vi "Get Kasli IP.vi"(8 "error in (no error)":errorcluster, 11 "Kasli Writer in":refnum<class "Kasli Writer.lvclass">) -> (0 "error out":errorcluster, 3 "Kasli Writer out":refnum<class "Kasli Writer.lvclass">)   [LabVIEW 2020, in "CIRCUS_uServices.lvlib" / "Kasli Listener and Writer.lvlib" / "Kasli Writer.lvclass"]
uses:
  Kasli Writer.lvclass
  C:/Users/marco/Documents/GitHub_Lab/CIRCUS/TALOS/TALOS_PPL.lvlibp/Ancestor/Ancestor/Ancestor.lvclass
  C:/Users/marco/Documents/GitHub_Lab/CIRCUS/TALOS/TALOS_PPL.lvlibp/Internal uServices/System uServices/TCP Writer/TCP Writer/TCP Writer.lvclass
  TALOS/TALOS_PPL.lvlibp/Ancestor/Ancestor/Read ID.vi
  TALOS/TALOS_PPL.lvlibp
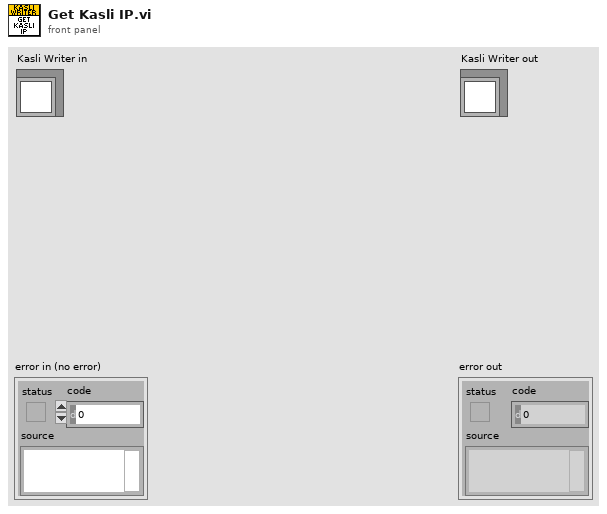
[diagram p1: front panel]
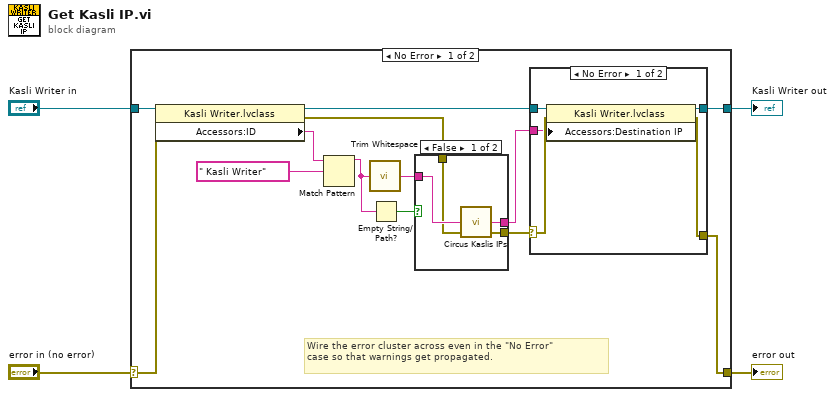
[diagram p0: block diagram]
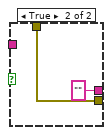
[diagram p3: hidden frame]
diagram:
  n1 = case shown="No Error" "error in (no error)" {
    selector: "error in (no error)" -> [w9 w32]
    tunnel: [w5 w32] -> w3
    tunnel: [w8 w31] -> w1
    tunnel: "Kasli Writer in" -> [w17 w31]
    frame No Error {
      # "Wire the error cluster across even in the \"No Error\"\ncase so that warnings get propagated."
      n2 = property class="Kasli Writer.lvclass"(reference=w17, error in=w9) -> (reference out=w16:refnum<class "Kasli Writer.lvclass">, error out=w10:errorcluster, "Accessors:ID"=w15:string)
      n3 = Match Pattern(string=w15, regular expression=" Kasli Writer") -> (before substring=w11:string)  [unwired: 1 in, 3 out]
      n4 = call <vilib>:"Trim Whitespace.vi"("string"=w11) -> ("trimmed string"=w12:string)  [unwired: 1 in]
      n5 = Empty String/Path?(string/path=w11) -> (empty?=w13:bool)
      n6 = case shown="False" w13 {
        tunnel: w12 -> [w28 _]
        tunnel: [w26 "" ("IP")] -> w7
        tunnel: [w25 w29] -> w6
        tunnel: w10 -> [w27 w29]
        frame False {
          n7 = call "Circus Kaslis IPs.vi"("error in (no error)"=w27, "ID"=w28) -> ("error out"=w25:errorcluster, "IP"=w26:string)  [unwired: 2 in]
        }
        frame True {
        }
      }
      n8 = case shown="No Error" w6 {
        selector: w6 -> [w22 w23]
        tunnel: w16 -> [w21 w24]
        tunnel: [w20 w24] -> w8
        tunnel: w7 -> [w19 _]
        tunnel: [w18 w23] -> w5
        frame No Error {
          n9 = property class="Kasli Writer.lvclass"(reference=w21, error in=w22, "Accessors:Destination IP"=w19) -> (reference out=w20:refnum<class "Kasli Writer.lvclass">, error out=w18:errorcluster)
        }
        frame Error {
        }
      }
    }
    frame Error {
    }
  }
  "error out" <- w3
  "Kasli Writer out" <- w1
